vi "Move_Z_Relative.vi"(2 "Pulse Number":i32=1000 min=1 max=500000, 3 "Residence time":i32=1, 4 "Axis Number":u8(ring)=1 items=["", "1", "2", "3", "4"], 5 "Port Number Z":i8=8 min=0) -> (0 "OK Done":bool=TRUE, 1 "String Received":string="OK\r\n")   [LabVIEW 2013]
panel:
  out "Received String2":string="R\r\n"
  out "Command String":string="A:1+P1000"
  # "Port Number 0=COM1"
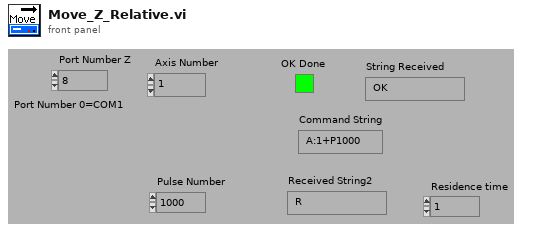
[diagram p1: front panel]
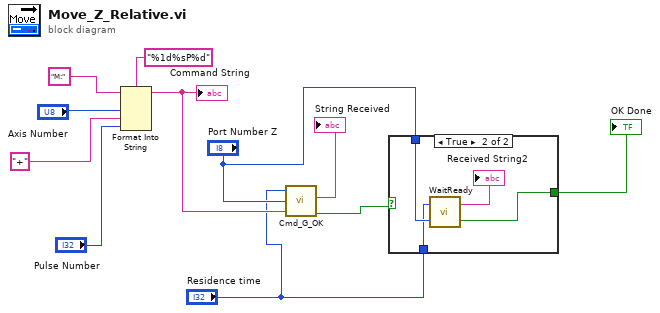
[diagram p0: block diagram]
diagram:
  n1 = Format Into String(format string="%1d%sP%d", initial string="M:", "Axis Number", "+", "Pulse Number") -> (resulting string=w7:string)  [unwired: 1 in, 1 out]
  "Command String" <- w7
  n2 = call "Cmd_G_OK.vi"("Residence time"="Residence time", "PortNumber"="Port Number Z", "Command String"=w7) -> ("Received String2"=→"String Received":string, "OK Done"=w4:bool)  [unwired: 2 out]
  n3 = case shown="True" w4 {
    selector: w4 -> [w12 _]
    tunnel: "Port Number Z" -> [_ w16]
    tunnel: [w12 w14] -> w3
    tunnel: "Residence time" -> [_ w13]
    frame False {
    }
    frame True {
      n4 = call "WaitReady.vi"("PortNumber"=w16, "Residence time in ms"=w13) -> ("OK Done"=w14:bool, "String Received"=→"Received String2":string)
    }
  }
  "OK Done" <- w3
